vi "Report Error.vi"(8 "error in (no error)":errorcluster) -> (0 "error out":errorcluster)   [LabVIEW 2021, in "XNET-CAN-Signal-Logger.lvlib"]
uses:
  XNET-CAN-Signal-Logger.lvlib
  Global Variables.vi
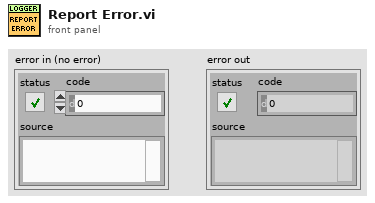
[diagram p1: front panel]
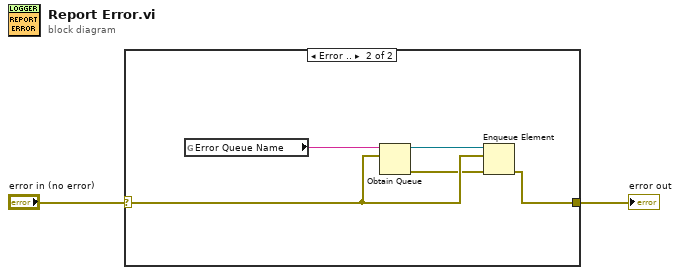
[diagram p0: block diagram]
diagram:
  n1 = case shown="Error .." "error in (no error)" {
    selector: "error in (no error)" -> [w3 w6]
    tunnel: [w3 w4] -> w1
    frame No Error {
    }
    frame Error {
      n2 = global read "Global Variables.vi" "Error Queue Name"() -> (w8:string)
      n3 = Obtain Queue(name (unnamed)=w8, element data type=w6) -> (queue out=w7:refnum<queue>, error out=w5:errorcluster)  [unwired: 3 in, 1 out]
      n4 = Enqueue Element(queue=w7, element=w6, error in (no error)=w5) -> (error out=w4:errorcluster)  [unwired: 1 in, 2 out]
    }
  }
  "error out" <- w1
